vi "subseq_around_index.vi"(8 "length around index 2":i32, 9 "index 2":i32, 10 "array length 2":i32, 11 "Array 3":i16[](array[numeric])) -> (0 "Array 2":i32[](array[numeric]))   [LabVIEW 2012]
uses:
  <vilib>/NXT/Dual Mode Library/prims/rotateArray/rotateArray_int.vi
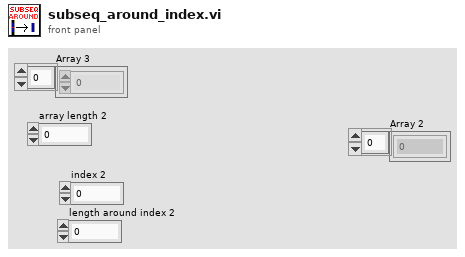
[diagram p1: front panel]
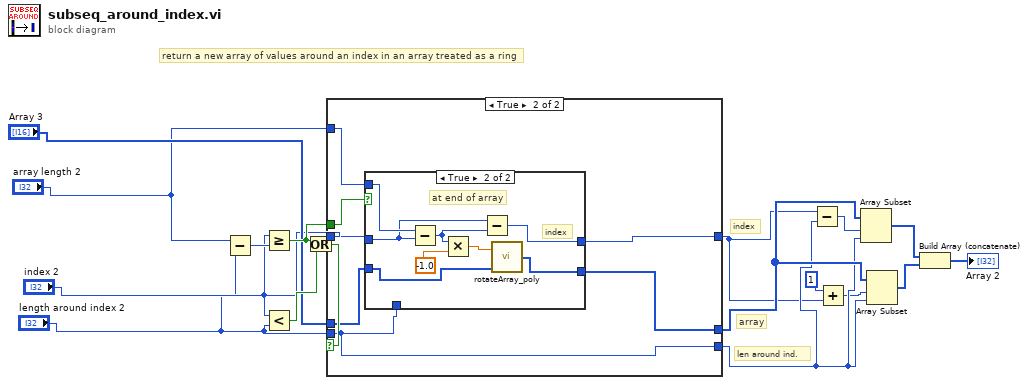
[diagram p0: block diagram]
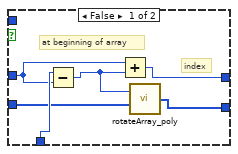
[diagram p3: hidden frame]
diagram:
  # "len around ind."
  # "array"
  # "index"
  # "return a new array of values around an index in an array treated as a ring"
  n1 = Subtract(x="array length 2", y="length around index 2") -> (x-y=w15:i32)
  n2 = Greater Or Equal?(x="index 2", y=w15) -> (x >= y?=w14:bool)
  n3 = Less?(x="index 2", y="length around index 2") -> (x < y?=w17:bool)
  n4 = Or(x=w14, y=w17) -> (x .or. y?=w16:bool)
  n5 = case shown="True" w16 {
    tunnel: w14 -> [_ w27]
    tunnel: "array length 2" -> [_ w24]
    tunnel: "length around index 2" -> [w19 w21]
    tunnel: "Array 3" -> [w20 w26]
    tunnel: "index 2" -> [w18 w25]
    tunnel: [w20 w22] -> w11
    tunnel: [w19 w21] -> w10
    tunnel: [w18 w23] -> w9
    frame False {
      # "in middle of array"
    }
    frame True {
      n6 = case shown="True" w27 {
        tunnel: w26 -> [w30 w38]
        tunnel: w25 -> [w32 w37]
        tunnel: w24 -> [_ w41]
        tunnel: [w29 w35] -> w23
        tunnel: w21 -> [w33 _]
        tunnel: [w28 w34] -> w22
        frame False {
          # "index"
          # "at beginning of array"
          n7 = Subtract(x=w33, y=w32) -> (x-y=w31:i32)
          n8 = Add(x=w32, y=w31) -> (x+y=w29:i32)
          n9 = call-poly <vilib>:"rotateArray_poly.vi"("Array"=w30, "n"=w31) -> ("rotated array"=w28:i32[])
        }
        frame True {
          # "index"
          # "at end of array"
          n10 = Subtract(x=w41, y=w37) -> (x-y=w36:i32)
          n11 = Multiply(x=w36, y=-1.0) -> (x*y=w39:dbl)
          n12 = Subtract(x=w37, y=w36) -> (x-y=w35:i32)
          n13 = call-poly <vilib>:"rotateArray_poly.vi"("Array"=w38, "n"=w39) -> ("rotated array"=w34:i32[])
        }
      }
    }
  }
  n14 = Subtract(x=w9, y=w10) -> (x-y=w12:i32)
  n15 = Add(x=1, y=w9) -> (x+y=w8:i32)
  n16 = Array Subset(array=w11, index=w12, length=w10) -> (w7:i32[])
  n17 = Array Subset(array=w11, index=w8, length=w10) -> (w6:i32[])
  n18 = Build Array (concatenate)(w7, w6) -> (→"Array 2":i32[])
